vi "LabBOT.vi"() -> ()   [LabVIEW 2020, in "Rover.lvlib"]
uses:
  Rover.lvlib
  LabBOT/LabBOT.lvclass
panel:
  out "error out":errorcluster
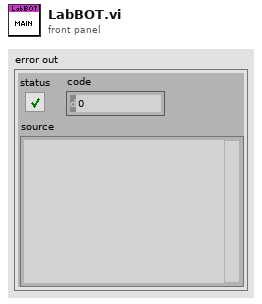
[diagram p1: front panel]
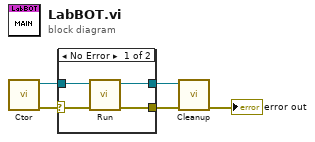
[diagram p0: block diagram]
diagram:
  n1 = call "Ctor.vi"() -> ("error out"=w5:errorcluster, "LabBOT out"=w4:refnum<class "LabBOT.lvclass">)  [unwired: 10 in]
  n2 = case shown="No Error" w5 {
    selector: w5 -> [w9 w11]
    tunnel: [w6 w11] -> w3
    tunnel: w4 -> [w8 w10]
    tunnel: [w7 w10] -> w2
    frame No Error {
      n3 = call "Run.vi"("error in (no error)"=w9, "LabBOT in"=w8) -> ("error out"=w6:errorcluster, "LabBOT out"=w7:refnum<class "LabBOT.lvclass">)  [unwired: 8 in]
    }
    frame Error {
    }
  }
  n4 = call "Cleanup.vi"("error in (no error)"=w3, "LabBOT in"=w2) -> ("error out"=→"error out":errorcluster)  [unwired: 9 in]
